vi "log_data.vi"(10 "Log data":bool, 11 "data":dynamicdata(waveform)) -> ()   [LabVIEW 2025]
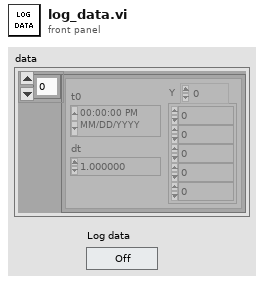
[diagram p1: front panel]
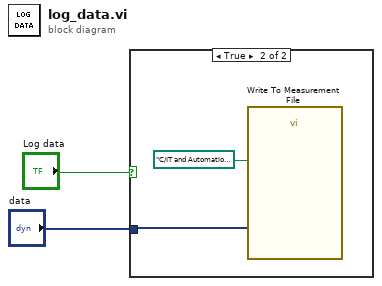
[diagram p0: block diagram]
diagram:
  n1 = case shown="True" "Log data" {
    tunnel: "data" -> [_ w4]
    frame False {
    }
    frame True {
      n2 = call "Write To Measurement File"("Signals"=w4, "Filename"=path "C:/IT and Automation master/2. semester/Industrial IT/DAQ and OPC Systems/industrial-it-daq-opc/LabView/temp_data.xlsx") -> ()  [unwired: 15 in, 3 out]
    }
  }
